vi "Init.vi"(6 "Allow Undefined Values (F)":bool, 8 "error in (no error)":errorcluster, 10 "Initial Options (Empty)":string[](array[string])) -> (0 "error out":errorcluster, 3 "Shared Config out":refnum<class "Shared Options.lvclass">)   [LabVIEW 2020, in "AutoComplete.lvlib" / "Shared Options.lvclass"]
doc: "Creates a Shared Options instance that can be used to have multiple autocomplete handled string inputs share options among each other. This makes it trivial to allow users to specify new options and share those new options among all autocompletes using the shared instanced."
uses:
  Shared Options.lvclass
  Options.ctl
  Shared Options.lvclass/Shared Options.ctl
  AutoComplete.lvlib
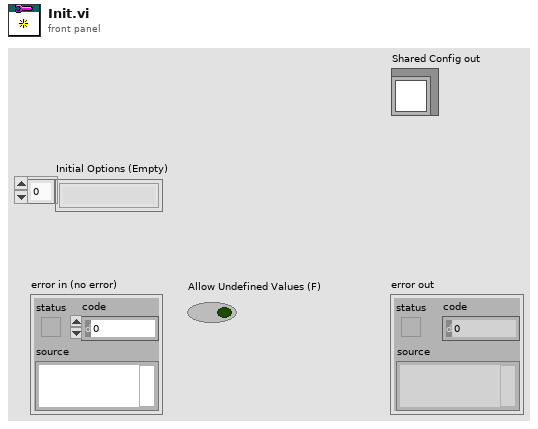
[diagram p1: front panel]
types:
  T1 = typedef "AutoComplete.lvlib/Options.ctl" = cluster{"Options":string[], "Allow Undefined Values":bool}
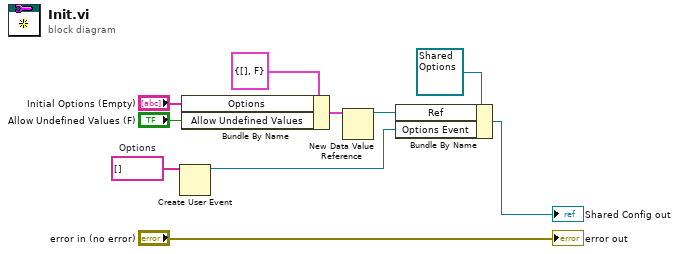
[diagram p0: block diagram]
diagram:
  w2 = string[] []  # Options
  n1 = Create User Event(user event datatype=w2) -> (user event=w1:refnum<user-event>)  [unwired: 1 in, 1 out]
  n2 = Bundle By Name(cluster=T1 {"Options"=[], "Allow Undefined Values"=FALSE} ("Cluster"), "Options"="Initial Options (Empty)", "Allow Undefined Values"="Allow Undefined Values (F)") -> (w7:T1)
  n3 = New Data Value Reference(data value=w7) -> (data value reference=w3:refnum<data-value>)  [unwired: 1 in, 1 out]
  n4 = Bundle By Name(cluster=refnum<class "Shared Options.lvclass"> refnum ("Shared Config in"), "Ref"=w3, "Options Event"=w1) -> (→"Shared Config out":refnum<class "Shared Options.lvclass">)
  "error out" <- "error in (no error)"
